vi "Voltage Parameters.vi"(0 "Data Management Control":T1, 5 "Capacitance Calculated Values":T2, 11 "Error In":errorcluster) -> (4 "Voltage Calculated Values":T3, 15 "Error Out":errorcluster)   [LabVIEW 2013]
uses:
  Controls/Data Management.ctl
  Controls/Capacitance Individual Calculated Values.ctl
  Controls/Voltage Calculated Values.ctl
panel:
  in  "Tab Control":enum32{"Inputs", "Outputs"}(tab)
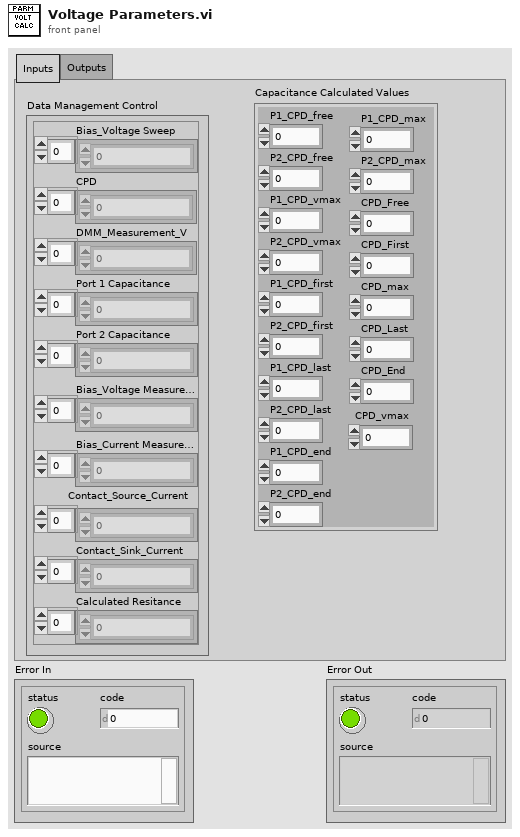
[diagram p1: front panel]
types:
  T1 = typedef "Data Management.ctl" = cluster{"Bias_Voltage Sweep":dbl[], "CPD":dbl[], "DMM_Measurement_V":dbl[], "Port 1 Capacitance":dbl[], "Port 2 Capacitance":dbl[], "Bias_Voltage Measurement":dbl[], "Bias_Current Measurement":dbl[], "Contact_Source_Current":dbl[], "Contact_Sink_Current":dbl[], "Calculated Resitance":dbl[]}
  T2 = typedef "Capacitance Individual Calculated Values.ctl" = cluster{"P1_CPD_free":dbl, "P2_CPD_free":dbl, "P1_CPD_vmax":dbl, "P2_CPD_vmax":dbl, "P1_CPD_first":dbl, "P2_CPD_first":dbl, "P1_CPD_last":dbl, "P2_CPD_last":dbl, "P1_CPD_end":dbl, "P2_CPD_end":dbl, "P1_CPD_max":dbl, "P2_CPD_max ":dbl, "CPD_Free":dbl, "CPD_First":dbl, "CPD_max":dbl, "CPD_Last":dbl, "CPD_End":dbl, "CPD_vmax":dbl}
  T3 = typedef "Voltage Calculated Values.ctl" = cluster{"P1_VPD_C":dbl, "P2_VPD_C":dbl, "P1_VPD_Rel_C":dbl, "P2_VPD_Rel_C":dbl}
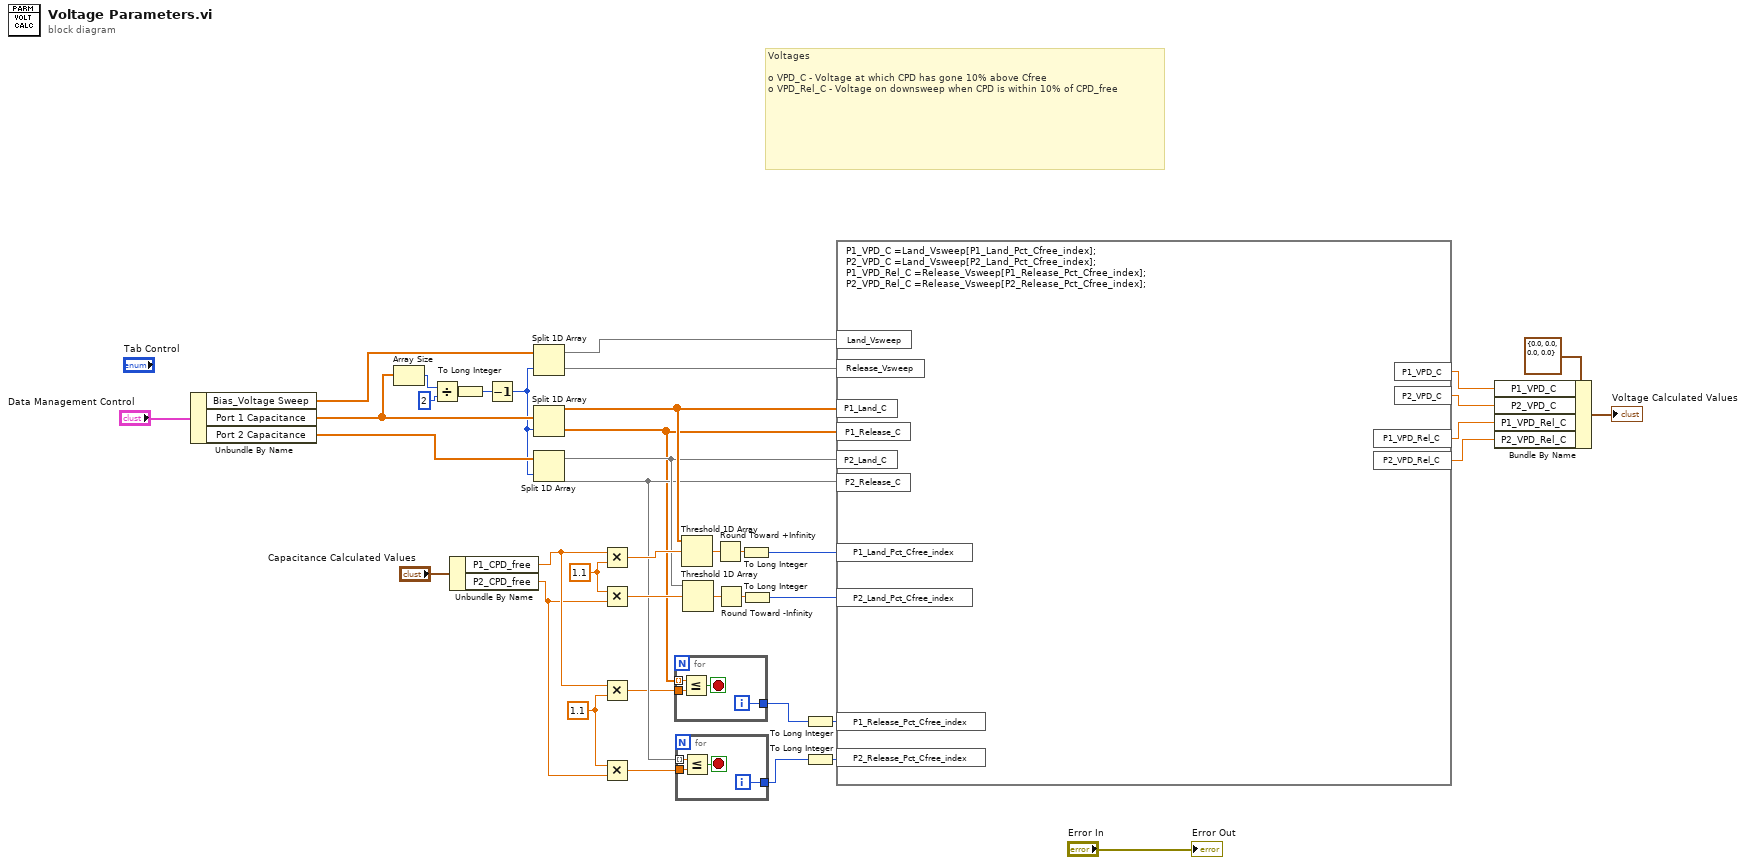
[diagram p0: block diagram]
diagram:
  w21 = 1.1 ("y")
  w27 = 1.1 ("y")
  # "Voltages\n\no\tVPD_C - Voltage at which CPD has gone 10% above Cfree\no\tVPD_Rel_C - Voltage on downsweep when CPD is within 10% of CPD_free"
  n1 = Unbundle By Name("Data Management Control") -> ("Bias_Voltage Sweep"=w16:dbl[], "Port 1 Capacitance"=w31:dbl[], "Port 2 Capacitance"=w30:dbl[])
  n2 = Array Size(array=w31) -> (size(s)=w35:i32)
  n3 = Divide(x=w35, y=2) -> (x/y=w33:dbl)
  n4 = Unbundle By Name("Capacitance Calculated Values") -> ("P1_CPD_free"=w20:dbl, "P2_CPD_free"=w19:dbl)
  n5 = To Long Integer(number=w33) -> (32bit integer=w32:i32)
  n6 = Decrement(x=w32) -> (x-1=w17:i32)
  n7 = Split 1D Array(array=w16, index=w17) -> (first subarray=w15:dbl[], second subarray=w14:dbl[])
  n8 = Split 1D Array(array=w31, index=w17) -> (first subarray=w29:dbl[], second subarray=w3:dbl[])
  n9 = Split 1D Array(array=w30, index=w17) -> (first subarray=w22:dbl[], second subarray=w6:dbl[])
  n10 = Multiply(x=w20, y=w27) -> (x*y=w28:dbl)
  n11 = Multiply(x=w27, y=w19) -> (x*y=w26:dbl)
  n12 = Multiply(x=w20, y=w21) -> (x*y=w2:dbl)
  n13 = Multiply(x=w21, y=w19) -> (x*y=w5:dbl)
  n14 = for {
    tunnel: [w45] -> w1
    tunnel: w3 -> [w44] mode=indexing
    tunnel: w2 -> [w43]
    i -> [w45]
    stop <- w42 stop-if-true
    n15 = Less Or Equal?(x=w44, y=w43) -> (x <= y?=w42:bool)
  }
  n16 = for {
    tunnel: [w49] -> w4
    tunnel: w6 -> [w48] mode=indexing
    tunnel: w5 -> [w47]
    i -> [w49]
    stop <- w46 stop-if-true
    n17 = Less Or Equal?(x=w48, y=w47) -> (x <= y?=w46:bool)
  }
  n18 = Threshold 1D Array(2:w28, 3:w29) -> (0:w39:dbl)  [unwired: 1 in]
  n19 = Threshold 1D Array(2:w26, 3:w22) -> (0:w37:dbl)  [unwired: 1 in]
  n20 = Round Toward +Infinity(x=w39) -> (ceil(x): smallest int >= x=w38:dbl)
  n21 = Round Toward -Infinity(1:w37) -> (0:w36:dbl)
  n22 = To Long Integer(number=w38) -> (32bit integer=w25:i32)
  n23 = To Long Integer(number=w36) -> (32bit integer=w24:i32)
  n24 = To Long Integer(number=w1) -> (32bit integer=w23:i32)
  n25 = To Long Integer(number=w4) -> (32bit integer=w18:i32)
  n26 = formula code="P1_VPD_C =Land_Vsweep[P1_Land_Pct_Cfree_index];\nP2_VPD_C =Land_Vsweep[P2_Land_Pct_Cfree_index];\nP1_VPD_Rel_C =Release_Vsweep[P1_Release_Pct_Cfree_index];\nP2_VPD_Rel_C =Release_Vsweep[P2_Release_Pct_Cfree_index];"("P1_Land_C"=w29, "P1_Release_C"=w3, "P2_Land_C"=w22, "P2_Release_C"=w6, "P1_Land_Pct_Cfree_index"=w25, "P2_Land_Pct_Cfree_index"=w24, "P1_Release_Pct_Cfree_index"=w23, "P2_Release_Pct_Cfree_index"=w18, "Land_Vsweep"=w15, "Release_Vsweep"=w14) -> ("P1_VPD_C"=w11:dbl, "P2_VPD_C"=w10:dbl, "P1_VPD_Rel_C"=w9:dbl, "P2_VPD_Rel_C"=w8:dbl)
  n27 = Bundle By Name(cluster=T3 {"P1_VPD_C"=0.0, "P2_VPD_C"=0.0, "P1_VPD_Rel_C"=0.0, "P2_VPD_Rel_C"=0.0} ("Voltage Calculated Values"), "P1_VPD_C"=w11, "P2_VPD_C"=w10, "P1_VPD_Rel_C"=w9, "P2_VPD_Rel_C"=w8) -> (→"Voltage Calculated Values":T3)
  "Error Out" <- "Error In"
